vi "Generate Segment Wildcard Regexp.vi"(11 "Options":T1) -> (3 "Segment Wildcard Regexp":string)   [LabVIEW 2020, in "Stream.lvlib" / "URLPattern.lvclass"]
uses:
  URLPattern.lvclass
  Pattern String Options.ctl
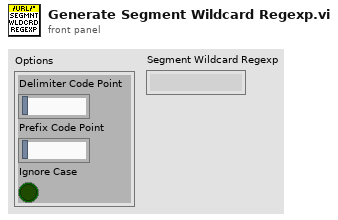
[diagram p1: front panel]
types:
  T1 = typedef "Stream.lvlib/URLPattern.lvclass/Pattern String Options.ctl" = cluster{"Delimiter Code Point":string, "Prefix Code Point":string, "Ignore Case":bool}
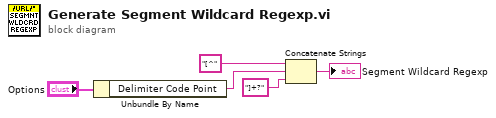
[diagram p0: block diagram]
diagram:
  n1 = Unbundle By Name("Options") -> ("Delimiter Code Point"=w3:string)
  n2 = Concatenate Strings("[^", w3, "]+?" ("string")) -> (→"Segment Wildcard Regexp":string)
